vi "Init.vi"(9 "Project:Active Project":refnum<vi>, 10 "NI.LV.Dialog Instance":refnum<vi>) -> (3 "_Template out":refnum<class "_Template.lvclass">)   [LabVIEW 2020, in "_Template.lvlib" / "_Template.lvclass"]
uses:
  _Template.lvclass
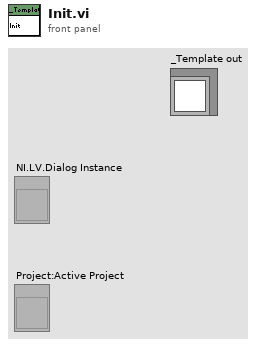
[diagram p1: front panel]
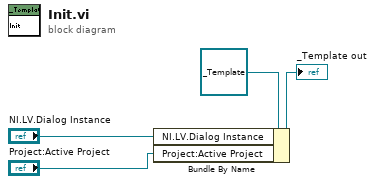
[diagram p0: block diagram]
diagram:
  n1 = Bundle By Name(cluster=refnum<class "_Template.lvclass"> refnum ("_Create From Template.lvlib:Script Strategy.lvlib:First Library Script Strategy.lvclass"), "NI.LV.Dialog Instance"="NI.LV.Dialog Instance", "Project:Active Project"="Project:Active Project") -> (→"_Template out":refnum<class "_Template.lvclass">)
